vi "Main Error.vi"(0 "All_ref":T1, 9 "Error Array":i32[](array[numeric]), 11 "error in (no error)":errorcluster, 12 "Error":bool) -> (10 "Error Array Out":i32[](array[numeric]), 14 "Error Out":bool, 15 "error out":errorcluster)   [LabVIEW 2015]
uses:
  0.GUI/Control/AllRef.ctl
panel:
  in  "中英":i32
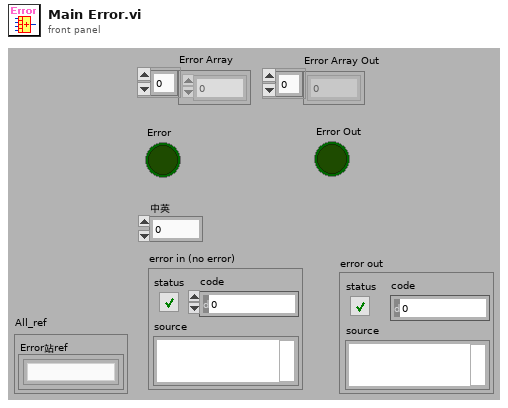
[diagram p1: front panel]
types:
  T1 = typedef "AllRef.ctl" = cluster{"Error站ref":T2}
  T2 = typedef "Error站_ref.ctl" = refnum<k1>
  T3 = typedef "Error站_Data.ctl" = cluster{"GUI":refnum<vi>, "Ready":bool, "Mode":T4, "Function":T5, "Porcedure in":u8, "空跑流程":bool, "異常處理":cluster{"Retry":bool, "Reset":bool, "Skip":bool}, "Message Array":i32[]}
  T4 = typedef "Error站_Mode.ctl" = enum8{"Idle", "Run", "Pause", "Err"}
  T5 = typedef "Error站_Function.ctl" = enum8{"預留"}
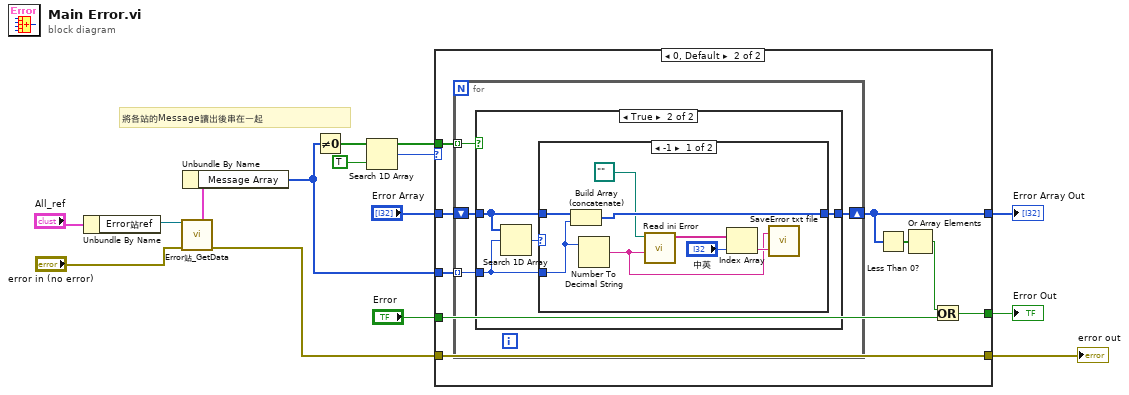
[diagram p0: block diagram]
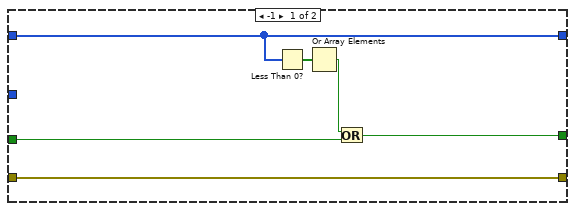
[diagram p2: hidden frame]
diagram:
  # "將各站的Message讀出後串在一起"
  n1 = Unbundle By Name("All_ref") -> ("Error站ref"=w6:T2)
  n2 = call "Error站_GetData.vi"("ref in"=w6, "error in"="error in (no error)") -> ("Data out"=w5:T3, "error out"=w2:errorcluster)  [unwired: 7 in, 5 out]
  n3 = Unbundle By Name(w5) -> ("Message Array"=w4:i32[])
  n4 = Not Equal To 0?(x=w4) -> (x != 0?=w12:bool[])
  n5 = Search 1D Array(1D array=w12, element=TRUE) -> (index of element=w13:i32)  [unwired: 1 in]
  n6 = case shown="0, Default" w13 {
    tunnel: w12 -> [_ w29]
    tunnel: "Error Array" -> [w18 w28]
    tunnel: w4 -> [_ w27]
    tunnel: [w18 w22] -> w10
    tunnel: "Error" -> [w17 w24]
    tunnel: [w16 w23] -> w8
    tunnel: w2 -> [w15 w21]
    tunnel: [w15 w21] -> w1
    frame -1 {
      n7 = Less Than 0?(x=w18) -> (x < 0?=w20:bool[])
      n8 = Or Array Elements(Boolean array=w20) -> (logical OR=w19:bool)
      n9 = Or(x=w19, y=w17) -> (x .or. y?=w16:bool)
    }
    frame 0, Default {
      n10 = for {
        tunnel: w29 -> [w33] mode=indexing
        shift-right: [w30] -> w22
        shift-left: w28 -> [w32]
        tunnel: w27 -> [w31] mode=indexing
        n11 = case shown="True" w33 {
          tunnel: w32 -> [w34 w37]
          tunnel: w31 -> [_ w36]
          tunnel: [w34 w35] -> w30
          frame False {
          }
          frame True {
            n12 = Search 1D Array(1D array=w37, element=w36) -> (index of element=w38:i32)  [unwired: 1 in]
            n13 = case shown="-1" w38 {
              tunnel: [w45 w47] -> w35
              tunnel: w37 -> [w46 w47]
              tunnel: w36 -> [w44 _]
              frame -1 {
                n14 = Build Array (concatenate)(w46, w44) -> (w45:i32[])
                n15 = Number To Decimal String(number=w44) -> (decimal integer string=w40:string)  [unwired: 1 in]
                n16 = call "Read ini Error.vi"("Error Code"=w40, "Error Code file path"=path "") -> ("Error message"=w43:string[])  [unwired: 9 in]
                n17 = Index Array(array=w43, index="中英") -> (element=w41:string)
                n18 = call "SaveError txt file.vi"("內容"=w41, "異常碼"=w40) -> ()  [unwired: 1 in]
              }
              frame 0, Default {
              }
            }
          }
        }
      }
      n19 = Less Than 0?(x=w22) -> (x < 0?=w26:bool[])
      n20 = Or Array Elements(Boolean array=w26) -> (logical OR=w25:bool)
      n21 = Or(x=w25, y=w24) -> (x .or. y?=w23:bool)
    }
  }
  "Error Array Out" <- w10
  "Error Out" <- w8
  "error out" <- w1
